vi "close.vi"(8 "error in (no error)":errorcluster, 11 "USB IO in":refnum<class "USB IO.lvclass">) -> (0 "error out":errorcluster, 3 "USB IO out":refnum<class "USB IO.lvclass">)   [LabVIEW 2025, in "USB IO.lvclass"]
uses:
  USB IO.lvclass
  USB IO.lvclass/USB IO.ctl
  <vilib>/DAQmx/write.llb/DAQmx Write (Digital 1D Bool NChan 1Samp 1Line).vi
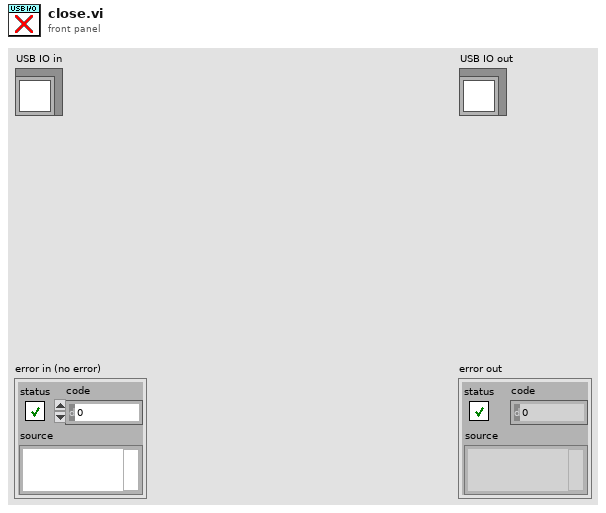
[diagram p1: front panel]
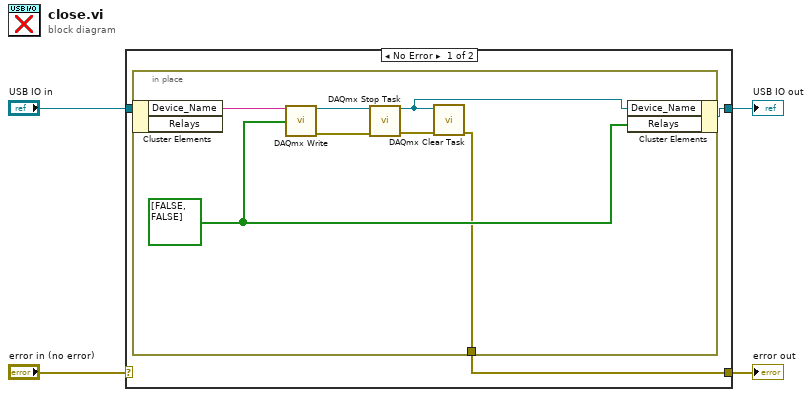
[diagram p0: block diagram]
diagram:
  n1 = case shown="No Error" "error in (no error)" {
    selector: "error in (no error)" -> [_ w16]
    tunnel: [w5 w16] -> w3
    tunnel: [w6 w15] -> w1
    tunnel: "USB IO in" -> [w7 w15]
    frame No Error {
      n2 = in-place {
        in-place-border: [w8] -> w5
        w10 = bool[] [FALSE, FALSE] ("data")
        n3 = in-place-cluster #1(w7) -> ("Device_Name"=w14:string)  [unwired: 1 out]
        n4 = call-poly <vilib>:"DAQmx Write.vi"("task/channels in"=w14, "data"=w10) -> ("task out"=w12:refnum<k21>, "error out"=w13:errorcluster)  [unwired: 11 in, 1 out]
        n5 = call <vilib>:"DAQmx Stop Task.vi"("task/channels in"=w12, "error in"=w13) -> ("task out"=w9:refnum<k21>, "error out"=w11:errorcluster)  [unwired: 12 in]
        n6 = call <vilib>:"DAQmx Clear Task.vi"("task in"=w9, "error in"=w11) -> ("error out"=w8:errorcluster)  [unwired: 13 in]
        n7 = in-place-cluster #1("Device_Name"=w9, "Relays"=w10) -> (w6:refnum<class "USB IO.lvclass">)
      }
    }
    frame Error {
    }
  }
  "error out" <- w3
  "USB IO out" <- w1
